vi "Measure.vi"(8 "error in (no error)":errorcluster, 9 "Variant":variant, 10 "Option":i32, 11 "Avantes in":refnum<class "Avantes.lvclass">) -> (0 "error out":errorcluster, 1 "Data Raw":T1(array[cluster]), 2 "Data":T1(array[cluster]), 3 "Avantes out":refnum<class "Avantes.lvclass">, 4 "Darkspec":T1(array[cluster]), 5 "Time":dbl[](array[numeric]), 6 "Starting Time":dbl)   [LabVIEW 2020, in "Avantes.lvclass"]
uses:
  <instrlib>/Classes/CCD/Avantes/Avantes.lvclass
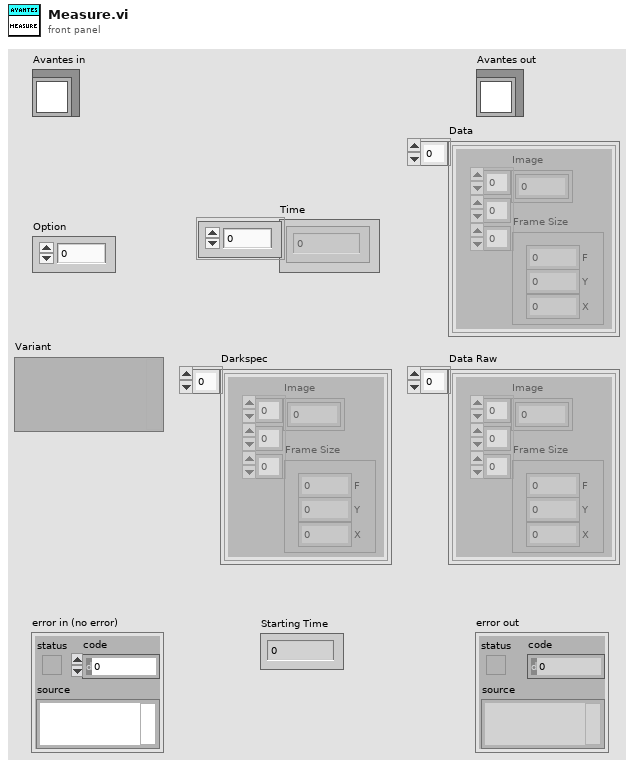
[diagram p1: front panel]
types:
  T1 = cluster{"Image":dbl[][][], "Frame Size":cluster{"F":i32, "Y":i32, "X":i32}}[]
  T2 = cluster{"Image":dbl[][][], "Frame Size":cluster{"F":i32, "Y":i32, "X":i32}}
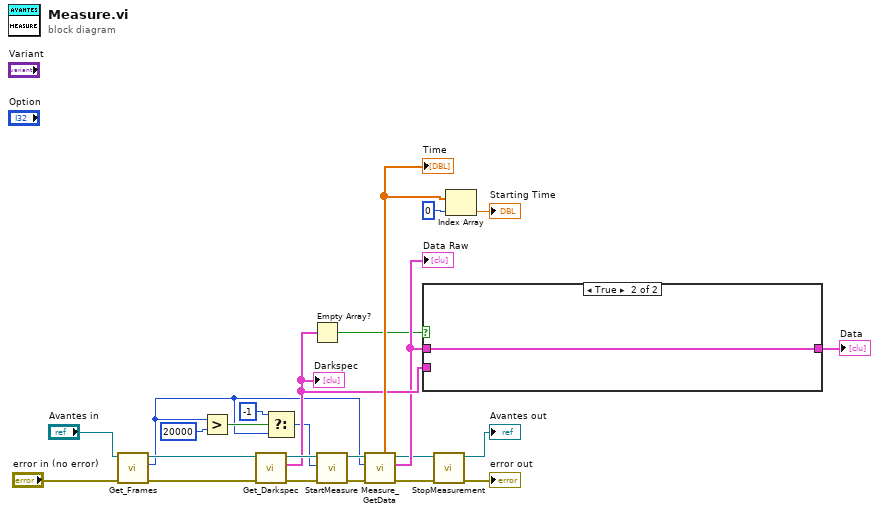
[diagram p0: block diagram]
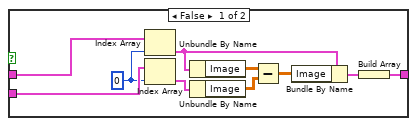
[diagram p2: hidden frame]
diagram:
  n1 = call-dynamic "Get_Frames.vi"("error in (no error)"="error in (no error)", "Avantes in"="Avantes in") -> ("error out"=w17:errorcluster, "Frames"=w1:i32, "Avantes out"=w16:refnum<class "Avantes.lvclass">)  [unwired: 7 in]
  n2 = Greater?(x=w1, y=20000) -> (0:w3:bool)
  n3 = call-dynamic "Get_Darkspec.vi"("error in (no error)"=w17, "Avantes in"=w16) -> ("error out"=w15:errorcluster, "Darkspec"=w11:T1, "Avantes out"=w14:refnum<class "Avantes.lvclass">)  [unwired: 7 in]
  "Darkspec" <- w11
  n4 = Select(t=-1 ("Frames"), s=w3, f=w1) -> (s? t:f=w2:i32)
  n5 = Empty Array?(array=w11) -> (empty?=w6:bool)
  n6 = call-dynamic "StartMeasure.vi"("error in (no error)"=w15, "Frames"=w2, "Avantes in"=w14) -> ("error out"=w13:errorcluster, "Avantes out"=w12:refnum<class "Avantes.lvclass">)  [unwired: 7 in]
  n7 = call-dynamic "Measure_GetData.vi"("error in (no error)"=w13, "SpectraCount"=w1, "Avantes in"=w12) -> ("error out"=w10:errorcluster, "Data_Raw"=w9:T1, "Avantes out"=w8:refnum<class "Avantes.lvclass">, "Time"=w20:dbl[])  [unwired: 5 in]
  "Time" <- w20
  "Data Raw" <- w9
  n8 = case shown="True" w6 {
    tunnel: w9 -> [w34 w35]
    tunnel: w11 -> [w33 _]
    tunnel: [w25 w35] -> w7
    frame False {
      w32 = 0 ("index")
      n9 = Index Array(array=w34, index=w32) -> (element=w28:T2)
      n10 = Index Array(array=w33, index=w32) -> (element=w31:T2)
      n11 = Unbundle By Name(w28) -> ("Image"=w30:dbl[][][])
      n12 = Unbundle By Name(w31) -> ("Image"=w29:dbl[][][])
      n13 = Subtract(x=w30, y=w29) -> (x-y=w27:dbl[][][])
      n14 = Bundle By Name(cluster=w28, "Image"=w27) -> (w26:T2)
      n15 = Build Array(w26) -> (w25:T1)
    }
    frame True {
    }
  }
  "Data" <- w7
  n16 = call-dynamic "StopMeasurement.vi"("error in (no error)"=w10, "Avantes in"=w8) -> ("error out"=→"error out":errorcluster, "Avantes out"=→"Avantes out":refnum<class "Avantes.lvclass">)  [unwired: 8 in]
  n17 = Index Array(array=w20, index=0) -> (element=→"Starting Time":dbl)
